vi "WS1021_MEMS Only Single Die AFS_Save Data_Ver1.0.vi"(0 "Header":string[](array[string]), 4 "File Name":string, 5 "error in (no error)":errorcluster, 6 "base path":path=path "C:/temp", 8 "Data In":string[][](array[string])) -> (12 "Final":string[][](array[string]), 19 "error out":errorcluster)   [LabVIEW 2017]
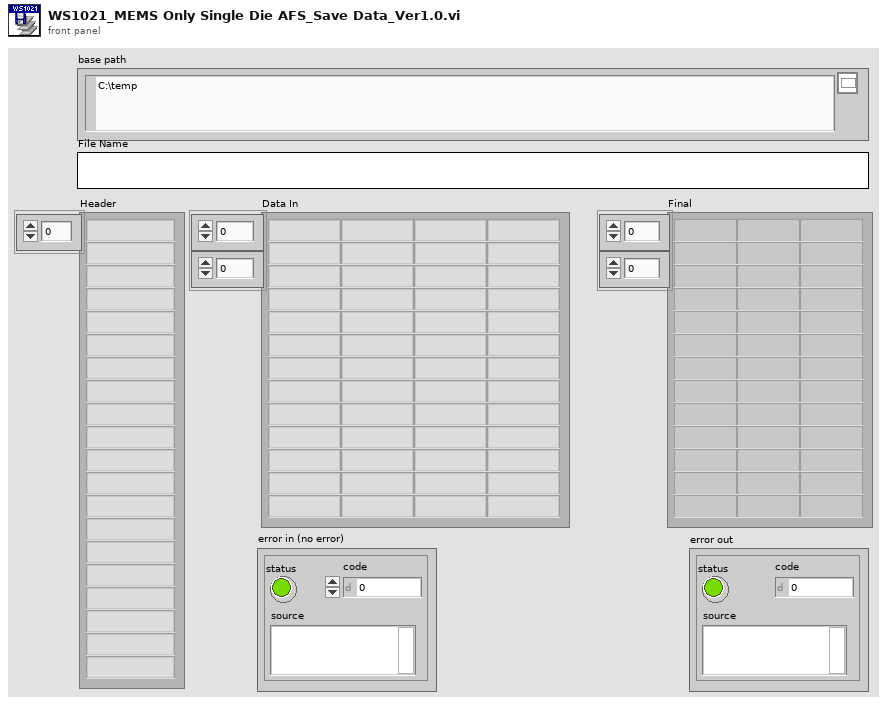
[diagram p1: front panel]
types:
  T1 = enum16{"open", "replace", "create", "open or create", "replace or create", "replace or create with confirmation"}
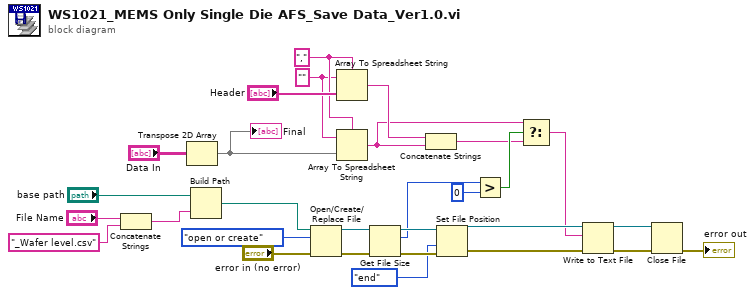
[diagram p0: block diagram]
diagram:
  w11 = "," ("delimiter (Tab)")
  w10 = "" ("format string")
  n1 = Concatenate Strings("File Name", "_Wafer level.csv" ("name or relative path")) -> (w4:string)
  n2 = Transpose 2D Array(2D array="Data In") -> (transposed array=w1:string[][])
  "Final" <- w1
  n3 = Build Path(base path="base path", name or relative path=w4) -> (appended path=w28:path)
  n4 = Open/Create/Replace File(file path (use dialog)=w28, error in="error in (no error)", operation (0:open)=T1."open or create") -> (refnum out=w25:refnum<file>, error out=w26:errorcluster)  [unwired: 3 in, 1 out]
  n5 = Array To Spreadsheet String(delimiter (Tab)=w11, array="Header", 3:w10) -> (spreadsheet string=w15:string)
  n6 = Array To Spreadsheet String(delimiter (Tab)=w11, array=w1, 3:w10) -> (spreadsheet string=w13:string)
  n7 = Get File Size(file=w25, error in=w26) -> (refnum out=w22:refnum<file>, size (in bytes)=w19:i64, 0:w24:errorcluster)
  n8 = Concatenate Strings(w15, w13) -> (w14:string)
  n9 = Set File Position(refnum=w22, from (0:start)=enum16{"start", "end", "current"}."end", error in=w24) -> (refnum out=w20:refnum<file>, error out=w21:errorcluster)  [unwired: 1 in]
  n10 = Greater?(x=w19, y=i64 0) -> (0:w17:bool)
  n11 = Select(t=w13, s=w17, f=w14) -> (s? t:f=w16:string)
  n12 = Write to Text File(file (use dialog)=w20, text=w16, error in=w21) -> (refnum out=w7:refnum<file>, error out=w8:errorcluster)  [unwired: 1 in, 1 out]
  n13 = Close File(refnum=w7, error in=w8) -> (error out=→"error out":errorcluster)  [unwired: 1 out]
